vi "get data.vi"(8 "error in (no error)":errorcluster, 11 "JSON in":string) -> (0 "error out":errorcluster, 1 "data array":string[](array[string]) caption="<JSON>Elements", 2 "Item Names":string[](array[string]), 3 "<JSON>":string[](array[string]))   [LabVIEW 2019]
uses:
  <vilib>/JDP Science/JSONtext/String Subset.vi
  <vilib>/JDP Science/JSONtext/support/Strip Quotes and Unescape.vi
  <vilib>/JDP Science/JSONtext/support/Unescape JSON string.vi
  <vilib>/JDP Science/JSONtext/Parsing/Parse Full Path or Item Name.vi
  <vilib>/JDP Science/JSONtext/Offset/Find Item Locations by Path.vi
  <vilib>/JDP Science/JSONtext/JSONtext.lvlib
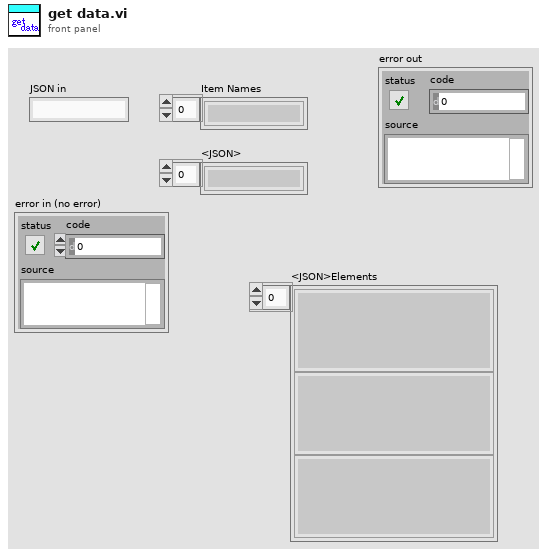
[diagram p1: front panel]
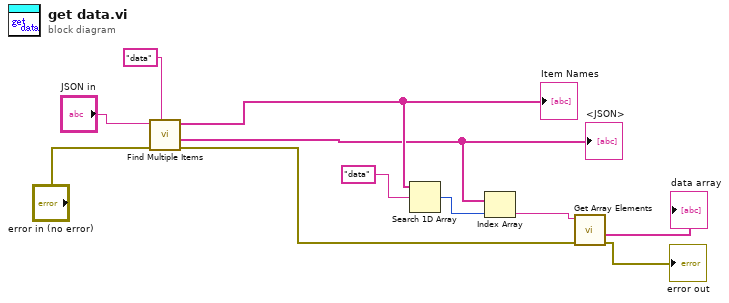
[diagram p0: block diagram]
diagram:
  n1 = call <vilib>:"Find Multiple Items.vi"("$Path or Item Name"="data", "error in (no error)"="error in (no error)", "JSON"="JSON in") -> ("error out"=w3:errorcluster, "<JSON>"=w6:string[], "Item Names"=w8:string[])  [unwired: 5 in, 1 out]
  "<JSON>" <- w6
  "Item Names" <- w8
  n2 = Search 1D Array(1D array=w8, element="data") -> (index of element=w5:i32)  [unwired: 1 in]
  n3 = Index Array(array=w6, index=w5) -> (element=w4:string)
  n4 = call <vilib>:"Get Array Elements.vi"("error in (no error)"=w3, "JSON"=w4) -> ("error out"=→"error out":errorcluster, "<JSON>"=→"data array":string[])  [unwired: 7 in, 1 out]
